vi "positionzuboundigrectangle.vi"(9 "Y Resolution":i32, 10 "X Resolution":i32, 11 "Position":cluster{"x":sgl, "y":sgl}) -> (3 "Cluster":cluster{dbl, dbl, dbl, dbl})   [LabVIEW 2014]
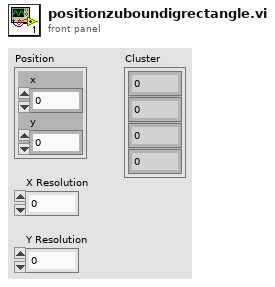
[diagram p1: front panel]
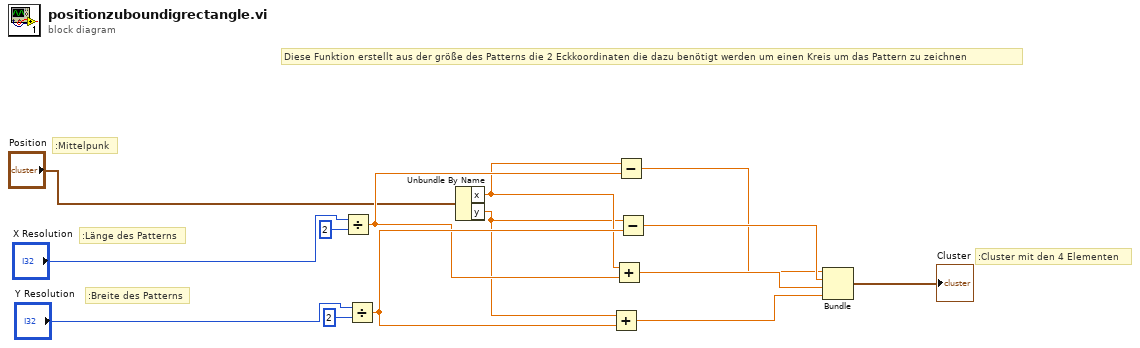
[diagram p0: block diagram]
diagram:
  # ":Cluster mit den 4 Elementen"
  # ":Breite des Patterns"
  # ":Länge des Patterns"
  # ":Mittelpunk"
  # "Diese Funktion erstellt aus der größe des Patterns die 2 Eckkoordinaten die dazu benötigt werden um einen Kreis um das Pattern zu zeichnen"
  n1 = Divide(x="X Resolution", y=2) -> (x/y=w13:dbl)
  n2 = Divide(x="Y Resolution", y=2) -> (x/y=w14:dbl)
  n3 = Unbundle By Name("Position") -> ("x"=w5:sgl, "y"=w4:sgl)
  n4 = Add(x=w4, y=w14) -> (x+y=w7:dbl)
  n5 = Add(x=w5, y=w13) -> (x+y=w6:dbl)
  n6 = Subtract(x=w5, y=w13) -> (x-y=w2:dbl)
  n7 = Subtract(x=w4, y=w14) -> (x-y=w3:dbl)
  n8 = Bundle(w2, w3, w6, w7) -> (→"Cluster":cluster{dbl, dbl, dbl, dbl})  [unwired: 1 in]
